vi "to string.vi"(8 "error in":errorcluster, 11 "fixed channel configuration in":refnum<class "ActiveFrontEndModule configuration.lvclass">) -> (0 "error out":errorcluster, 1 "data":string, 2 "version":string, 3 "fixed channel configuration out":refnum<class "ActiveFrontEndModule configuration.lvclass">)   [LabVIEW 2017, in "ActiveFrontEndModule configuration.lvclass"]
doc: "Provides an interface for saving a module configuration to a file or other serialized data source. It is recommended that all children of this class store data in two sets--data required for its own initialization, and any data required for parent initialization--and that each implementation uses the <b>Call Parent Method</b> primitive to serialize parent information.\nNI Tag Bus Module Framework 1.0.3.43\nNI Systems Engineering"
uses:
  ActiveFrontEndModule configuration.lvclass
  ActiveFrontEndModule configuration.lvclass/ActiveFrontEndModule configuration.ctl
  <vilib>/NI/JSON Support for LabVIEW/JSON Data Classes/JSON Object/New JSON Object (Empty).vi
  <vilib>/NI/JSON Support for LabVIEW/JSON Data Classes/JSON Object/Insert Key Value Pair.vi
  <vilib>/NI/JSON Support for LabVIEW/JSON Data Classes/JSON Object/Insert Key Value Pair (Single).vi
  <vilib>/NI/DCAF/Tag Editor Core/control module/configuration/control module configuration.lvclass
  <vilib>/NI/JSON Support for LabVIEW/JSON Data Classes/JSON Object/Set Object Parameters XNode/Set Object Parameters.xnode
  <vilib>/NI/JSON Support for LabVIEW/JSON Data Classes/JSON Datatype/JSON Null.lvclass
  <vilib>/NI/JSON Support for LabVIEW/JSON Data Classes/JSON Object/JSON Object.lvclass
  <vilib>/NI/Configuration Framework/serializable configuration/NISE_CEF_serializable configuration.lvclass
  <vilib>/NI/JSON Support for LabVIEW/JSON Data Classes/JSON Helper/JSON Helper.lvclass
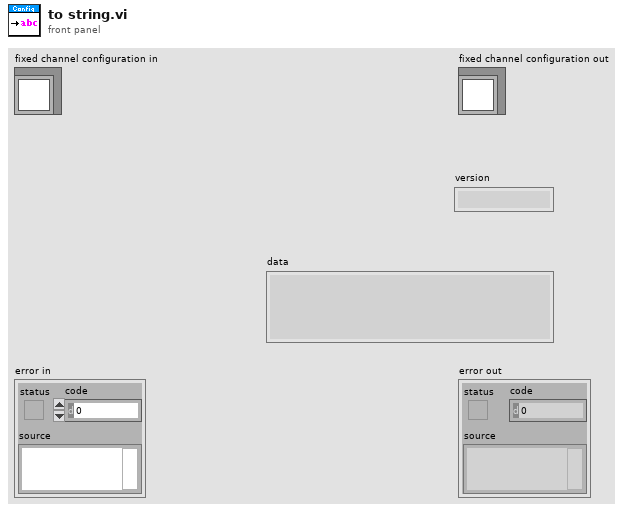
[diagram p1: front panel]
types:
  T1 = typedef "ActiveFrontEnd.lvlib/Parameters.ctl" = cluster{"VDCLink_setpt":sgl, "VDCLinkRampRate":sgl, "Q_setpt":sgl, "Pf_setpt":sgl, "Mode":T2, "perturbance_amp":sgl, "perturbance_freq":sgl, "dT":sgl}
  T2 = typedef "ActiveFrontEnd.lvlib/Mode.ctl" = enum16{"Q Control", "Pf Control"}
  T3 = typedef "ActiveFrontEnd.lvlib/PI_Settings.ctl" = cluster{"gains":T4, "output range":T5, "PI_state":enum8{"idle", "normal", "manual", "perturbance"}, "reset":bool, "manual":sgl}
  T4 = typedef "niFpgaPID_PIGains.ctl" = cluster{"proportional gain":sgl, "integral gain":sgl}
  T5 = typedef "niFpgaPID_OutputRange.ctl" = cluster{"output high (Inf)":sgl, "output low (-Inf)":sgl}
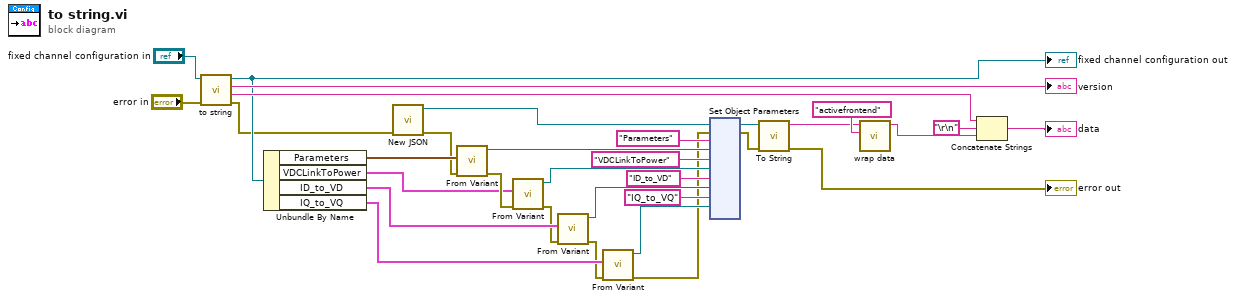
[diagram p0: block diagram]
diagram:
  n1 = call-parent "to string.vi"("error in"="error in", "fixed channel configuration in"="fixed channel configuration in") -> ("error out"=w9:errorcluster, "data"=w28:string, "version"=→"version":string, "fixed channel configuration out"=w25:refnum<class "ActiveFrontEndModule configuration.lvclass">)  [unwired: 6 in]
  "fixed channel configuration out" <- w25
  n2 = Unbundle By Name(w25) -> ("Parameters"=w24:T1, "VDCLinkToPower"=w22:T3, "ID_to_VD"=w21:T3, "IQ_to_VQ"=w19:T3)
  n3 = call-poly <vilib>:"New JSON.vi"("error in (no error)"=w9) -> ("error out"=w8:errorcluster, "JSON Object out"=w7:refnum<class "JSON Object.lvclass">)  [unwired: 9 in]
  n4 = call <vilib>:"From Variant.vi"("error in (no error)"=w8, "Variant"=w24) -> ("error out"=w23:errorcluster, "JSON out"=w17:refnum<class "JSON Null.lvclass">)  [unwired: 8 in]
  n5 = call <vilib>:"From Variant.vi"("error in (no error)"=w23, "Variant"=w22) -> ("error out"=w20:errorcluster, "JSON out"=w16:refnum<class "JSON Null.lvclass">)  [unwired: 8 in]
  n6 = call <vilib>:"From Variant.vi"("error in (no error)"=w20, "Variant"=w21) -> ("error out"=w18:errorcluster, "JSON out"=w15:refnum<class "JSON Null.lvclass">)  [unwired: 8 in]
  n7 = call <vilib>:"From Variant.vi"("error in (no error)"=w18, "Variant"=w19) -> ("error out"=w5:errorcluster, "JSON out"=w14:refnum<class "JSON Null.lvclass">)  [unwired: 8 in]
  n8 = xnode "Set Object Parameters"("key"="Parameters", "key"="VDCLinkToPower", "key"="ID_to_VD", "key"="IQ_to_VQ", "parameter"=w17, "parameter"=w16, "parameter"=w15, "parameter"=w14, "JSON Object In"=w7, "error in"=w5) -> ("JSON Object Out"=w6:refnum<class "JSON Object.lvclass">, "error out"=w4:errorcluster)  [unwired: 4 out]
  n9 = call-dynamic "To String.vi"("error in (no error)"=w4, "JSON Object in"=w6) -> ("error out"=→"error out":errorcluster, "String"=w3:string)  [unwired: 8 in]
  n10 = call <vilib>:"wrap data.vi"("identifier"="activefrontend", "data to wrap"=w3) -> ("wrapped data"=w2:string)  [unwired: 9 in]
  n11 = Concatenate Strings(w28, "\r\n", w2) -> (→"data":string)
